vi "setTestMode.vi"(8 "error in (no error)":errorcluster, 10 "Test":bool, 11 "Game in":refnum<class "Game.lvclass">) -> (0 "error out":errorcluster, 3 "Game out":refnum<class "Game.lvclass">)   [LabVIEW 2021, in "Game.lvclass"]
uses:
  Game.lvclass
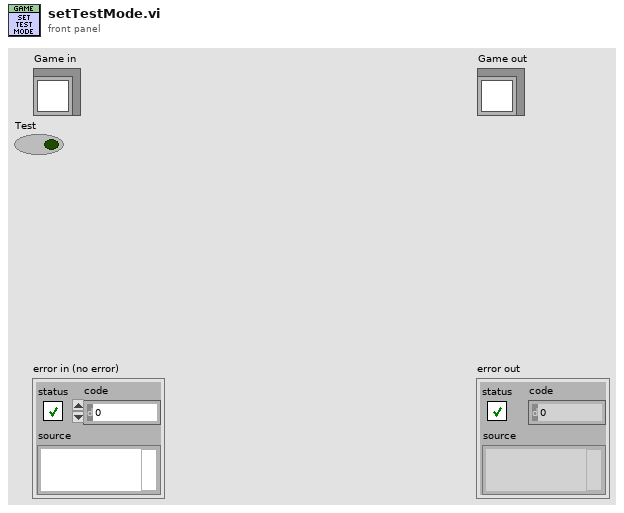
[diagram p1: front panel]
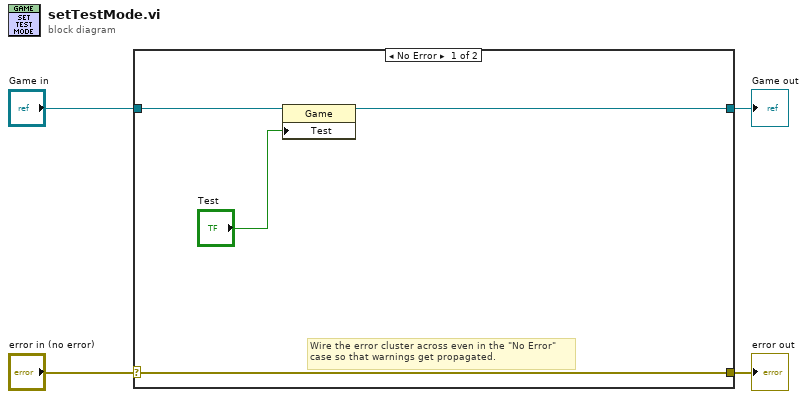
[diagram p0: block diagram]
diagram:
  n1 = case shown="No Error" "error in (no error)" {
    selector: "error in (no error)" -> [w8 w10]
    tunnel: [w8 w10] -> w3
    tunnel: [w6 w9] -> w1
    tunnel: "Game in" -> [w7 w9]
    frame No Error {
      # "Wire the error cluster across even in the \"No Error\"\ncase so that warnings get propagated."
      n2 = property class="Game"(reference=w7, "Test"="Test") -> (reference out=w6:refnum<class "Game.lvclass">)  [unwired: 1 in, 1 out]
    }
    frame Error {
    }
  }
  "error out" <- w3
  "Game out" <- w1
